vi "Add Single.vi"(0 "UI in":refnum<class "Assembly Run.lvclass">, 2 "Routine":T1=enum."Release Syringe", 4 "Fixture":T2, 5 "error in (no error)":errorcluster, 6 "Settings":T3, 7 "Module Size":bool) -> (14 "UI out":refnum<class "Assembly Run.lvclass">, 19 "error out":errorcluster)   [LabVIEW 2016, in "Assembly Run.lvclass"]
uses:
  Assembly Run.lvclass
  Routine/Settings.ctl
  Workspace/Fixture Enum.ctl
  Routine/Routine Enum.ctl
  Routine/Routine.lvclass
  Workspace/Fixture.lvclass
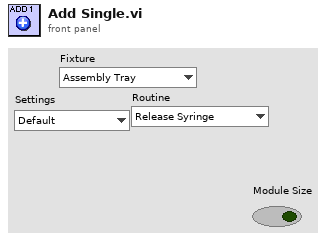
[diagram p1: front panel]
types:
  T1 = typedef "Routine.lvclass/Routine Enum.ctl" = enum16{"Primary Pick Up", "Pick Up All", "Put Down Secondary", "Put Down All", "Release Syringe", "Secondary Pick Up", "Secure Syringe", "Dispense on Plate", "Dispense on Kapton", "Dispense on Sensor"}
  T2 = typedef "Fixture.lvclass/Fixture Enum.ctl" = enum16{"Assembly Tray", "Syringe Space", "Component", "Pick Up Tool", "Current Position"}
  T3 = typedef "Routine.lvclass/Settings.ctl" = enum16{"Default", "Custom"}
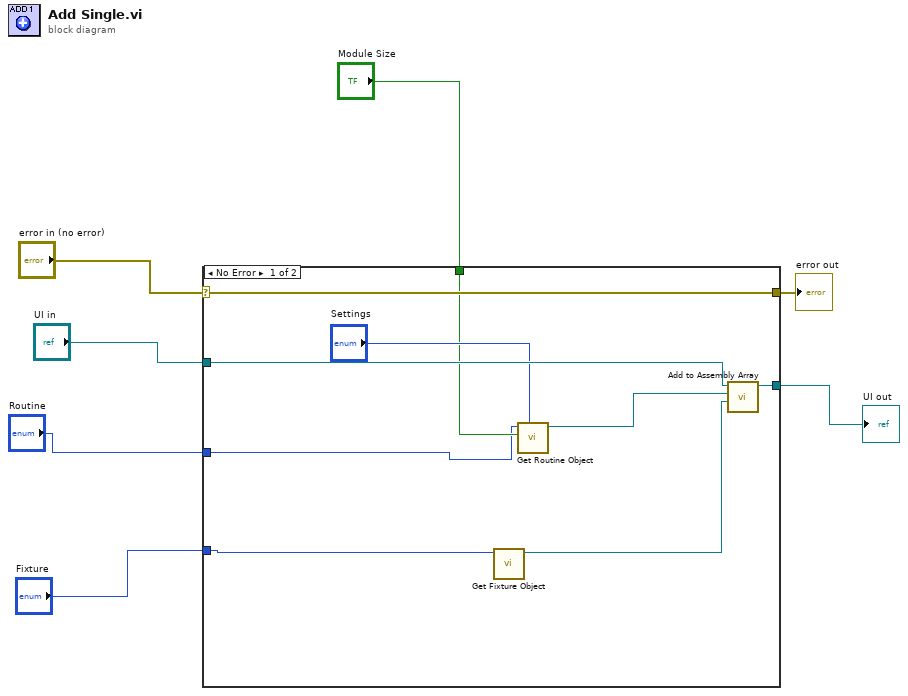
[diagram p0: block diagram]
diagram:
  n1 = case shown="No Error" "error in (no error)" {
    selector: "error in (no error)" -> [w16 w18]
    tunnel: [w16 w18] -> w6
    tunnel: "UI in" -> [w15 w17]
    tunnel: [w14 w17] -> w4
    tunnel: "Fixture" -> [w11 _]
    tunnel: "Module Size" -> [w9 _]
    tunnel: "Routine" -> [w8 _]
    frame No Error {
      n2 = call "Get Fixture Object.vi"("Fixture"=w11) -> ("Workspace.lvclass"=w10:refnum<class "Fixture.lvclass">)  [unwired: 8 in, 2 out]
      n3 = call "Get Routine Object.vi"("Settings"="Settings", "6 Inch"=w9, "Routine"=w8) -> ("Routine out"=w13:refnum<class "Routine.lvclass">)  [unwired: 7 in, 1 out]
      n4 = call "Add to Assembly Array.vi"("Workspace In"=w10, "Routine In"=w13, "Assembly Run in"=w15) -> ("Assembly Run out"=w14:refnum<class "Assembly Run.lvclass">)  [unwired: 7 in, 1 out]
    }
    frame Error {
    }
  }
  "error out" <- w6
  "UI out" <- w4
